vi "forward-propagation.vi"(6 "Number of Examples":i32, 7 "X":dbl[][](array[numeric]), 8 "b2":dbl[](array[numeric]), 9 "W2":dbl[][](array[numeric]), 10 "b1":dbl[](array[numeric]), 11 "W1":dbl[][](array[numeric])) -> (0 "A2":dbl[][](array[numeric]), 1 "Z2":dbl[][](array[numeric]), 2 "A1":dbl[][](array[numeric]), 3 "Z1":dbl[][](array[numeric]))   [LabVIEW 2023]
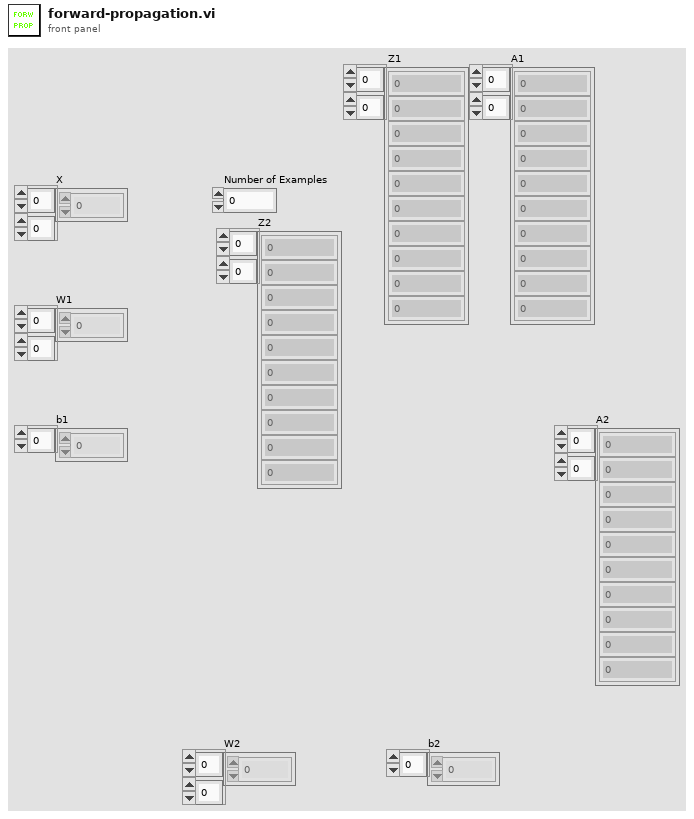
[diagram p1: front panel]
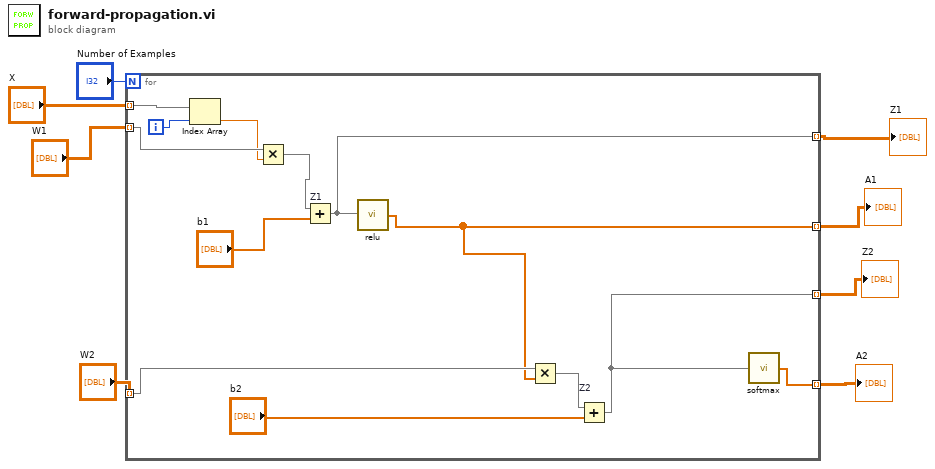
[diagram p0: block diagram]
diagram:
  n1 = for {
    N: "Number of Examples" -> [_]
    tunnel: "X" -> [w21] mode=indexing
    tunnel: "W1" -> [w19] mode=indexing
    tunnel: "W2" -> [w16] mode=indexing
    tunnel: [w14] -> w2 mode=indexing
    tunnel: [w13] -> w3 mode=indexing
    tunnel: [w12] -> w1 mode=indexing
    tunnel: [w11] -> w4 mode=indexing
    i -> [w20]
    n2 = Index Array(array=w21, index=w20) -> (element=w18:dbl)
    n3 = Multiply(x=w19, y=w18) -> (x*y=w17:dbl[])
    n4 = Add "Z1"(x=w17, y="b1") -> (x+y=w13:dbl[])
    n5 = call "relu.vi"("Array"=w13) -> (">=0"=w14:dbl[])
    n6 = Multiply(x=w16, y=w14) -> (x*y=w15:dbl[])
    n7 = Add "Z2"(x=w15, y="b2") -> (x+y=w12:dbl[])
    n8 = call "softmax.vi"("Array"=w12) -> ("softmax"=w11:dbl[])
  }
  "A2" <- w4
  "Z1" <- w3
  "A1" <- w2
  "Z2" <- w1
